vi "Actor Core.vi"(8 "error in":errorcluster, 11 "UIActor in":refnum<class "UIActor.lvclass">) -> (0 "error out":errorcluster, 3 "Actor out":refnum<class "Actor.lvclass">)   [LabVIEW 2015, in "UIActor.lvlib" / "UIActor.lvclass"]
doc: "(<B>Filename</B>: Actor Framework.lvlib:Actor.lvclass:Actor Core.vi)\n\nReceives messages to the actor, reacts to them, and initiates any error handling that may shut the actor down.\n\nDescendant classes may override this VI to append parallel tasks for the actor to complete while it handles messages. Overrides use the Call Parent Method node."
uses:
  UIActor.lvclass
  <vilib>/ActorFramework/Actor/Actor.lvclass
  MainControlsActor/MainControlsActor/MainControlsActor.lvclass
  MP3SearchActor/MP3SearchActor/MP3SearchActor.lvclass
  SongLibraryBrowserActor/SongLibraryBrowserActor/SongLibraryBrowserActor.lvclass
  SongPlayerActor/SongPlayerActor/SongPlayerActor.lvclass
panel:
  in  "Main UI":enum32{"Main", "Debug"}(tab)
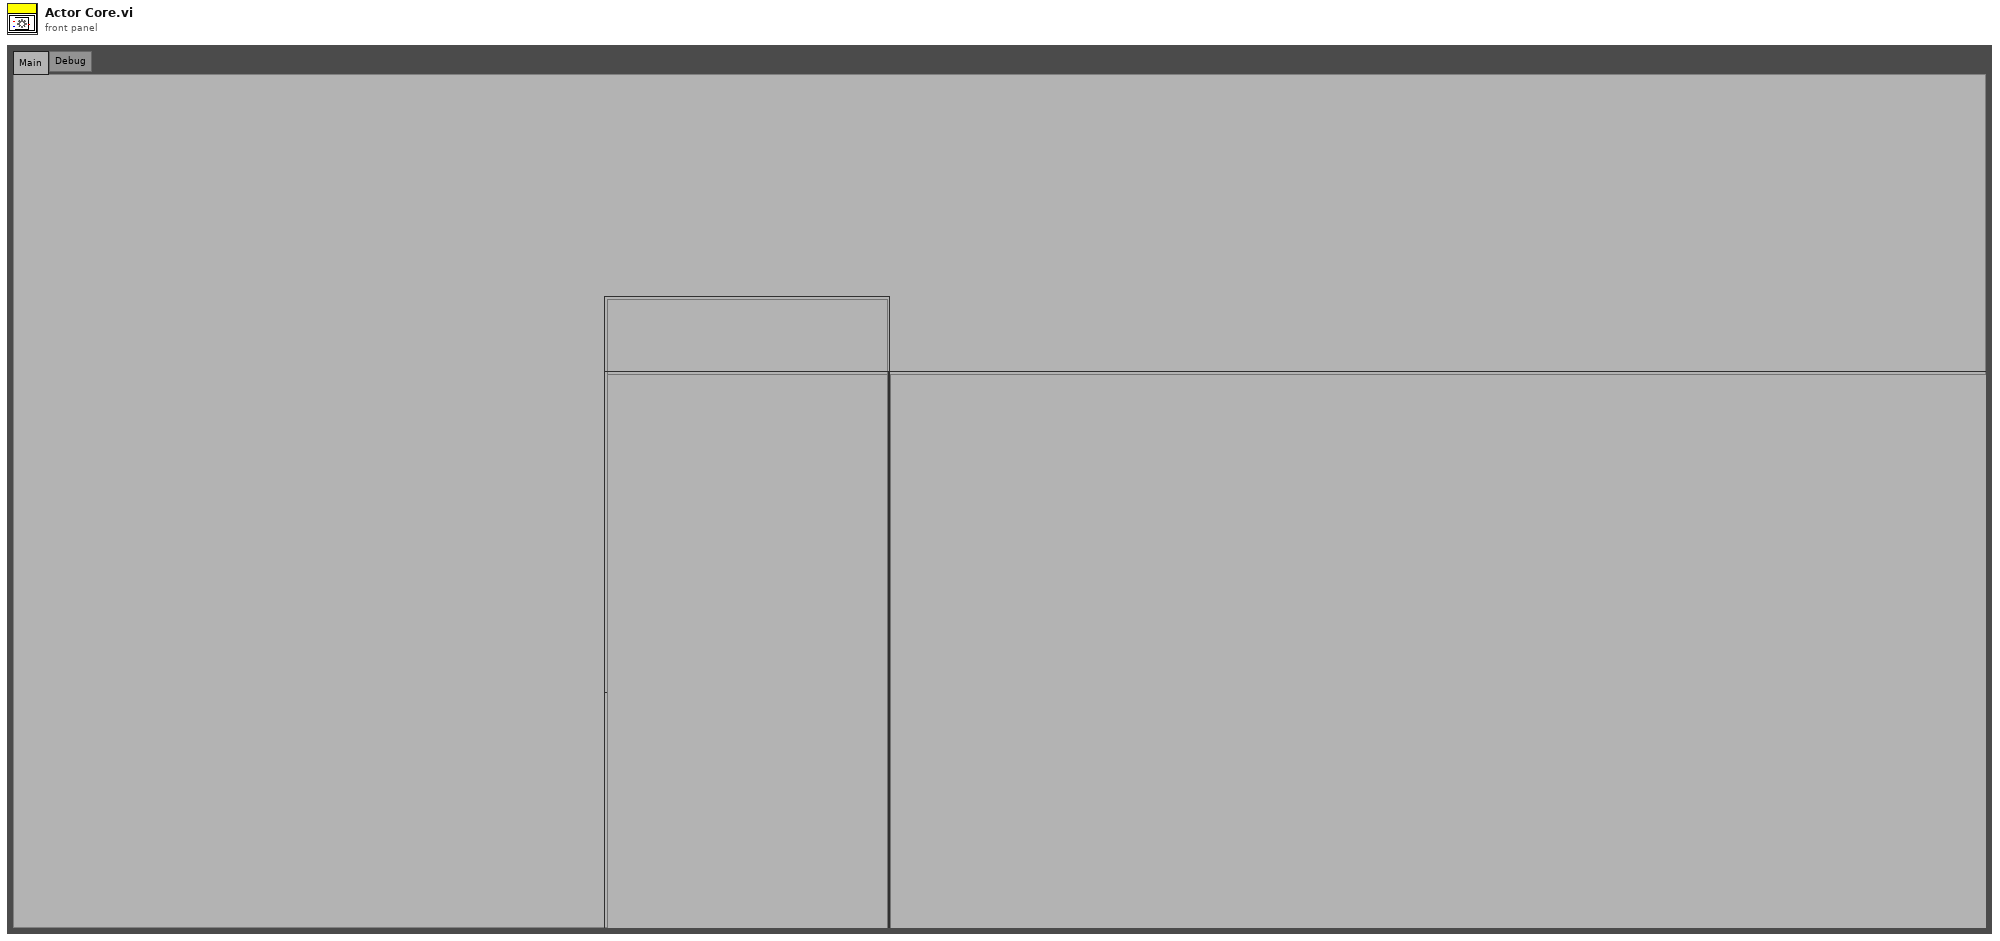
[diagram p1: front panel]
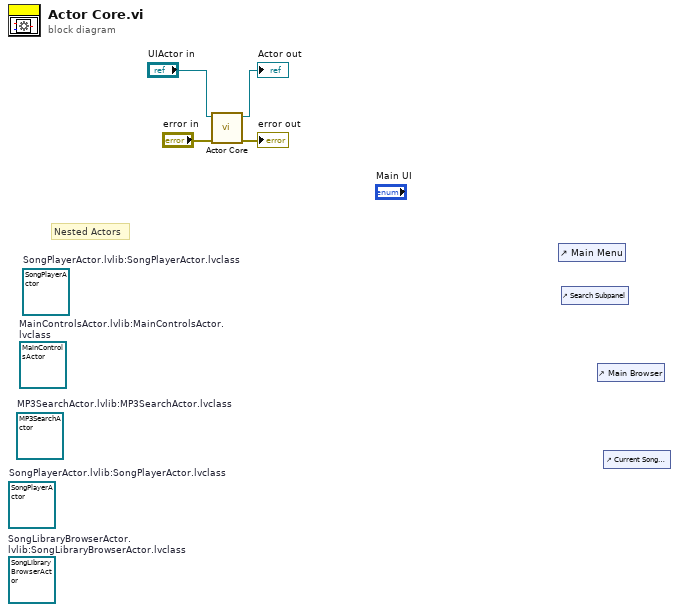
[diagram p0: block diagram]
diagram:
  (unwired) refnum<class "SongPlayerActor.lvclass"> refnum  # SongPlayerActor.lvlib:SongPlayerActor.lvclass
  (unwired) refnum<class "SongLibraryBrowserActor.lvclass"> refnum  # SongLibraryBrowserActor.lvlib:SongLibraryBrowserActor.lvclass
  (unwired) refnum<class "SongPlayerActor.lvclass"> refnum  # SongPlayerActor.lvlib:SongPlayerActor.lvclass
  (unwired) refnum<class "MP3SearchActor.lvclass"> refnum  # MP3SearchActor.lvlib:MP3SearchActor.lvclass
  (unwired) refnum<class "MainControlsActor.lvclass"> refnum  # MainControlsActor.lvlib:MainControlsActor.lvclass
  # "Nested Actors"
  n1 = call-parent "Actor Core.vi"("error in"="error in", "Actor in"="UIActor in") -> ("error out"=→"error out":errorcluster, "Actor out"=→"Actor out":refnum<class "Actor.lvclass">)  [unwired: 8 in]
  n2 = control-ref of="Main Menu"() -> ()  [unwired: 1 out]
  n3 = control-ref of="Search Subpanel"() -> ()  [unwired: 1 out]
  n4 = control-ref of="Main Browser"() -> ()  [unwired: 1 out]
  n5 = control-ref of="Current Song Subpanel"() -> ()  [unwired: 1 out]
